vi "WriteToMeasurementRing.vi"(8 "error in (no error)":errorcluster, 11 "SiemensDigitalEnergyMeter in":refnum<class "SiemensDigitalEnergyMeter.lvclass">) -> (0 "error out":errorcluster, 3 "SiemensDigitalEnergyMeter out":refnum<class "SiemensDigitalEnergyMeter.lvclass">)   [LabVIEW 2018, in "SensorPlugins.lvlib" / "SiemensDigitalEnergyMeter.lvclass"]
uses:
  SiemensDigitalEnergyMeter.lvclass
  C:/Program Files (x86)/National Instruments/LabVIEW 2018/user.lib/NIST/BaseClasses/BasePlugin_class/BasePlugin.lvclass
  TypeDefinitions/SiemensDigitalEnergyMeterControls.ctl
  <userlib>/NIST/BaseClasses/BasePlugin_class/BasePlugin.lvclass/BasePlugin.ctl
  <userlib>/NIST/BaseClasses/BasePlugin_class/Accessors/Read PluginIniFilePath.vi
  <vilib>/Utility/config.llb/NI_LVConfig.lvlib
panel:
  in  "Text Ring":u16(ring)
  out "Siemens Digital Energy Meter":T1 {"Measurement(s)" items=["kWh System"=4000, "kVARh System"=4007, "kVAh System"=4010, "kVA System"=4012, "Volts L1 to L2"=4018, "Volts L2 to L3"=4019, "Volts L1 to L2"=4020, "Line Frequency"=4021, "kW L1"=4028, "kW L2"=4029, "kW L3"=4030, "kVAR L1"=4037, "kVAR L2"=4038, "kVAR L3"=4039, "kVA L1"=4046, "kVA L2"=4047, "kVA L3"=4048, "Apparent PF L1"=4052, "Apparent PF L2"=4053, "Apparent PF L3"=4054, "Amps L1"=4055, "Amps L2"=4056, "Amps L3"=4057, "Volts L1 to Neutral"=4058, "Volts L2 to Neutral"=4059, "Volts L3 to Neutral"=4060, "Firmware Major Revision"=4068, "Firmware Minor Revision "=4069, "Model Number "=4200, "Serial Number"=4205, "Hardware ID"=4510]}
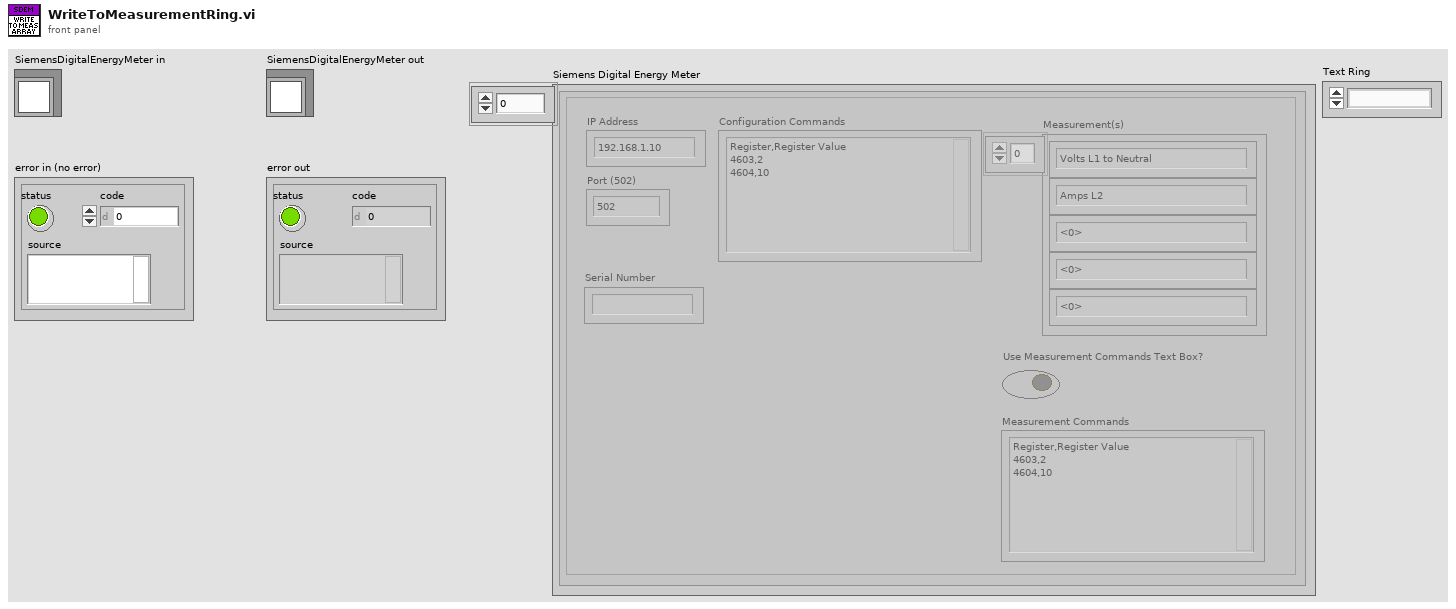
[diagram p1: front panel]
types:
  T1 = typedef "SensorPlugins.lvlib/SiemensDigitalEnergyMeter.lvclass/SiemensDigitalEnergyMeterControls.ctl" = cluster{"Measurement(s)":u16[], "IP Address":string, "Port (502)":u16, "Configuration Commands":string, "Use Measurement Commands Text Box?":bool, "Measurement Commands":string, "Connected?":bool, "Serial Number":string}[]
  T2 = typedef "NI_LVConfig.lvlib/Config Data RefNum.ctl" = refnum<k1>
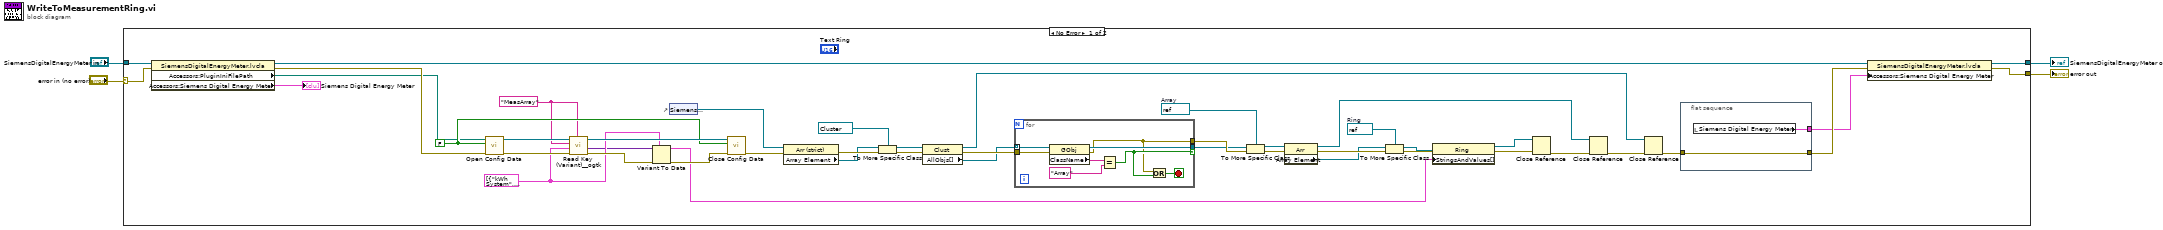
[diagram p0: block diagram]
diagram:
  n1 = case shown="No Error" "error in (no error)" {
    selector: "error in (no error)" -> [w49 w62]
    tunnel: [w35 w62] -> w3
    tunnel: [w47 w61] -> w1
    tunnel: "SiemensDigitalEnergyMeter in" -> [w50 w61]
    frame No Error {
      w24 = refnum<vi> refnum  # Ring
      w27 = refnum<vi> refnum  # Array
      w36 = "MeasArray" ("section")
      w41 = cluster{"String":string, "Value":u16}[] [{"String"="kWh System", "Value"=4000}, {"String"="kVARh System", "Value"=4007}, {"String"="kVAh System", "Value"=4010}, {"String"="kVA System", "Value"=4012}, {"String"="Volts L1 to L2", "Value"=4018}, {"String"="Volts L2 to L3", "Value"=4019}, {"String"="Volts L1 to L2", "Value"=4020}, {"String"="Line Frequency", "Value"=4021}, {"String"="kW L1", "Value"=4028}, {"String"="kW L2", "Value"=4029}, {"String"="kW L3", "Value"=4030}, {"String"="kVAR L1", "Value"=4037}, {"String"="kVAR L2", "Value"=4038}, {"String"="kVAR L3", "Value"=4039}, {"String"="kVA L1", "Value"=4046}, {"String"="kVA L2", "Value"=4047}, {"String"="kVA L3", "Value"=4048}, {"String"="Apparent PF L1", "Value"=4052}, {"String"="Apparent PF L2", "Value"=4053}, {"String"="Apparent PF L3", "Value"=4054}, {"String"="Amps L1", "Value"=4055}, {"String"="Amps L2", "Value"=4056}, {"String"="Amps L3", "Value"=4057}, {"String"="Volts L1 to Neutral", "Value"=4058}, {"String"="Volts L2 to Neutral", "Value"=4059}, {"String"="Volts L3 to Neutral", "Value"=4060}, {"String"="Firmware Major Revision", "Value"=4068}, {"String"="Firmware Minor Revision ", "Value"=4069}, {"String"="Model Number ", "Value"=4200}, {"String"="Serial Number", "Value"=4205}, {"String"="Hardware ID", "Value"=4510}] ("Array 3")
      w39 = FALSE ("create file if necessary (T)")
      n2 = property class="SiemensDigitalEnergyMeter.lvcla"(reference=w50, error in=w49) -> (reference out=w48:refnum<class "SiemensDigitalEnergyMeter.lvclass">, error out=w38:errorcluster, "Accessors:PluginIniFilePath"=w37:path, "Accessors:Siemens Digital Energy Meter"=→"Siemens Digital Energy Meter":T1)
      n3 = call <vilib>:"Open Config Data.vi"("error in (no error)"=w38, "create file if necessary (T)"=w39, "configuration file path"=w37) -> ("error out"=w46:errorcluster, "refnum"=w45:T2)  [unwired: 6 in, 1 out]
      n4 = call <userlib>:"Read Key (Variant)__ogtk.vi"("section"=w36, "error in (no error)"=w46, "type"=w41, "key (optional)"=w36, "refnum"=w45) -> ("error out"=w43:errorcluster, "key-value"=w40:variant, "refnum out"=w44:T2)  [unwired: 3 in, 1 out]
      n5 = Variant To Data(error in=w43, type=w41, Variant=w40) -> (data=w19:cluster{"String":string, "Value":u16}[], error out=w42:errorcluster)
      n6 = control-ref of="Siemens Digital Energy Meter"() -> (w33:refnum<vi>)
      n7 = call <vilib>:"Close Config Data.vi"("error in (no error)"=w42, "write file if changed (T)"=w39, "refnum"=w44) -> ("error out"=w34:errorcluster)  [unwired: 7 in, 1 out]
      n8 = property class="Arr (strict)"(reference=w33, error in=w34) -> (error out=w32:errorcluster, "Array Element"=w31:refnum<vi>)  [unwired: 1 out]
      n9 = To More Specific Class(target class=refnum<vi> refnum ("Text Ring"), reference=w31, error in=w32) -> (specific class reference=w28:refnum<vi>, error out=w29:errorcluster)
      n10 = property class="Clust"(reference=w28, error in=w29) -> (reference out=w6:refnum<vi>, error out=w9:errorcluster, "AllObjs[]"=w7:refnum<vi>[])
      n11 = for {
        tunnel: w7 -> [w58] mode=indexing
        tunnel: [w57] -> w5 if=w52
        tunnel: w9 -> [w54]
        tunnel: [w51] -> w8
        stop <- w53 stop-if-true
        n12 = property class="GObj"(reference=w58, error in=w54) -> (reference out=w57:refnum<vi>, error out=w51:errorcluster, "ClassName"=w56:string)
        n13 = Equal?(x=w56, y="Array" ("ClassName")) -> (x = y?=w52:bool)
        n14 = Or(x=w51, y=w52) -> (x .or. y?=w53:bool)
      }
      n15 = To More Specific Class(target class=w27, reference=w5, error in=w8) -> (specific class reference=w25:refnum<vi>, error out=w26:errorcluster)
      n16 = property class="Arr"(reference=w25, error in=w26) -> (reference out=w11:refnum<vi>, error out=w23:errorcluster, "Array Element"=w22:refnum<vi>)
      n17 = To More Specific Class(target class=w24, reference=w22, error in=w23) -> (specific class reference=w20:refnum<vi>, error out=w21:errorcluster)
      n18 = property class="Ring"(reference=w20, error in=w21, "StringsAndValues[]"=w19) -> (reference out=w17:refnum<vi>, error out=w18:errorcluster)
      n19 = Close Reference(reference=w17, error in (no error)=w18) -> (error out=w14:errorcluster)
      n20 = Close Reference(reference=w11, error in (no error)=w14) -> (error out=w13:errorcluster)
      n21 = Close Reference(reference=w6, error in (no error)=w13) -> (error out=w12:errorcluster)
      n22 = flat-sequence {
        tunnel: [w60] -> w16
        tunnel: [w59] -> w15
        tunnel: w12 -> [w60]
        frame #0 {
          n23 = local read "Siemens Digital Energy Meter"() -> (w59:T1)
        }
      }
      n24 = property class="SiemensDigitalEnergyMeter.lvcla"(reference=w48, error in=w16, "Accessors:Siemens Digital Energy Meter"=w15) -> (reference out=w47:refnum<class "SiemensDigitalEnergyMeter.lvclass">, error out=w35:errorcluster)
    }
    frame Error {
    }
  }
  "error out" <- w3
  "SiemensDigitalEnergyMeter out" <- w1
